vi "FGV Limit.vi"(5 "Limit":bool, 9 "action":enum16{"set", "get"}(ring)) -> (6 "Limit":bool)   [LabVIEW 2014, in "FH 55.lvlib"]
uses:
  FH 55.lvlib
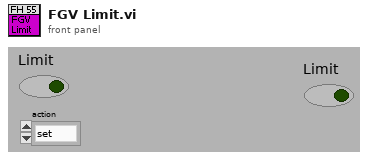
[diagram p1: front panel]
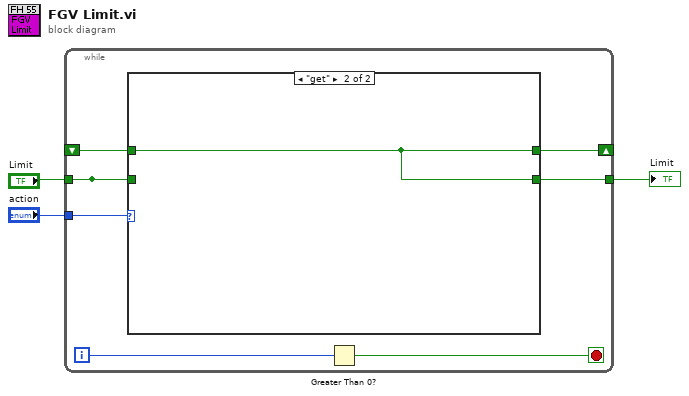
[diagram p0: block diagram]
diagram:
  n1 = while {
    tunnel: "Limit" -> [w9]
    tunnel: [w9] -> _
    shift-right: [w7] -> _
    shift-left: _ -> [w10]
    tunnel: [w8] -> w1
    tunnel: "action" -> [w4]
    i -> [w6]
    stop <- w5 stop-if-true
    n2 = case shown="\"get\"" w4 {
      tunnel: w10 -> [_ w12]
      tunnel: w9 -> [w11 _]
      tunnel: [w11 w12] -> w8
      tunnel: [w11 w12] -> w7
      frame "set", Default {
      }
      frame "get" {
      }
    }
    n3 = Greater Than 0?(x=w6) -> (x > 0?=w5:bool)
  }
  "Limit" <- w1
